vi "Disconnect.vi"(8 "error in":errorcluster, 11 "DAQ970 in":refnum<class "DAQ970.lvclass">) -> (0 "error out":errorcluster, 3 "DAQ970 out":refnum<class "DAQ970.lvclass">)   [LabVIEW 2019, in "DAQ970.lvlib" / "DAQ970.lvclass"]
uses:
  Library/DAQ970.lvclass
  Library/DAQ970.lvclass/DAQ970.ctl
  <instrlib>/Keysight DAQ970/Keysight DAQ970.lvlib
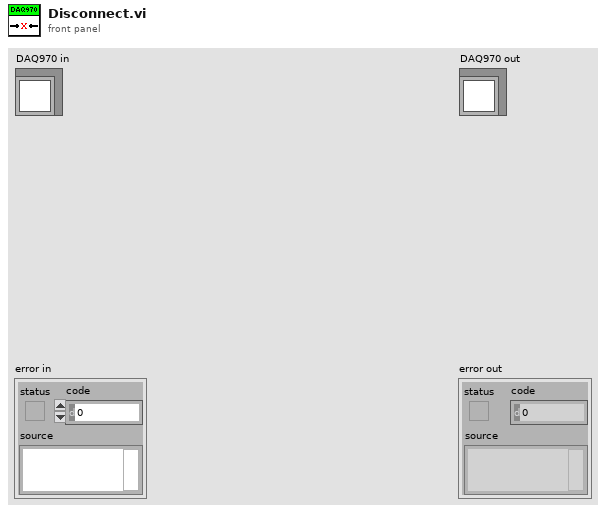
[diagram p1: front panel]
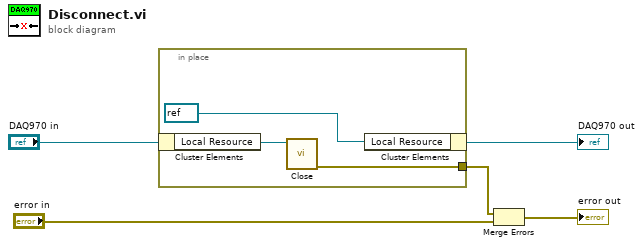
[diagram p0: block diagram]
diagram:
  n1 = in-place {
    in-place-border: [w6] -> w4
    n2 = in-place-cluster #1("DAQ970 in") -> ("Local Resource"=w8:refnum<k15>)
    n3 = call <instrlib>:"Close.vi"("instrument handle"=w8) -> ("error out"=w6:errorcluster)  [unwired: 10 in]
    n4 = in-place-cluster #1("Local Resource"=refnum<k15> refnum) -> (→"DAQ970 out":refnum<class "DAQ970.lvclass">)
  }
  n5 = Merge Errors(w4, "error in") -> (→"error out":errorcluster)
